vi "写入属性.vi"(6 "tdms文件":refnum<k34>, 7 "组名称输入（无标题）":string, 8 "错误输入（无错误）":errorcluster, 11 "数据属性":T1) -> (0 "错误输出":errorcluster, 4 "tdms文件输出":refnum<k34>, 5 "组名称输出":string)   [LabVIEW 2021]
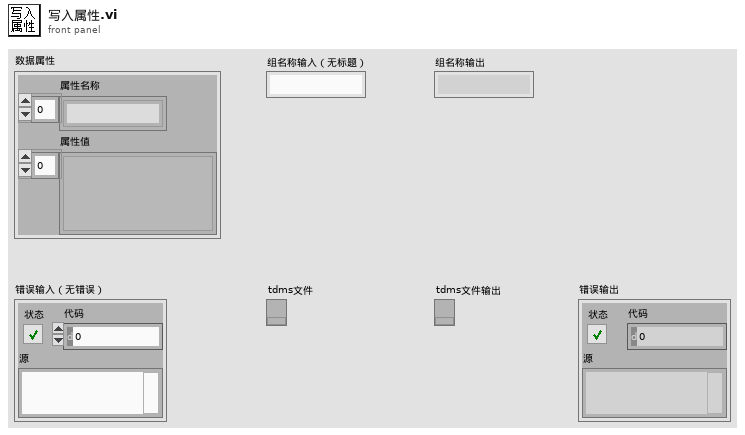
[diagram p1: front panel]
types:
  T1 = typedef "数据属性.ctl" = cluster{"属性名称":string[], "属性值":variant[]}
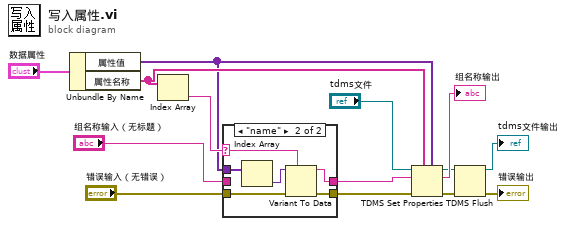
[diagram p0: block diagram]
diagram:
  n1 = Unbundle By Name("数据属性") -> ("属性值"=w1:variant[], "属性名称"=w7:string[])
  n2 = Index Array(array=w7) -> (element=w6:string)  [unwired: 1 in]
  n3 = case shown="\"name\"" w6 {
    selector: w6 -> [_ w17]
    tunnel: w1 -> [_ w22]
    tunnel: "组名称输入（无标题）" -> [w16 _]
    tunnel: [w16 w20] -> w4
    tunnel: "错误输入（无错误）" -> [w15 w19]
    tunnel: [w15 w18] -> w2
    frame Default {
    }
    frame "name" {
      n4 = Index Array(array=w22) -> (element=w21:variant)  [unwired: 1 in]
      n5 = Variant To Data(error in=w19, type=w17, Variant=w21) -> (data=w20:string, error out=w18:errorcluster)
    }
  }
  n6 = TDMS Set Properties(5:w1, 7:w7, 8:w2, 10:w4, 11:"tdms文件") -> (0:w11:errorcluster, 2:→"组名称输出":string, 3:w9:refnum<k34>)  [unwired: 1 in, 1 out]
  n7 = TDMS Flush(4:w11, 7:w9) -> (0:→"错误输出":errorcluster, 3:→"tdms文件输出":refnum<k34>)
